vi "subvi_SerialRead.vi"(4 "tf_exit(Refnum)":refnum<vi>, 5 "Error In":errorcluster, 6 "error_out(Refnum)":refnum<vi>, 7 "baud_rate":u32=9600, 8 "tb_read_datetime(Refnum)":refnum<vi>, 9 "tb_read(Refnum)":refnum<vi>, 10 "tf_status(Refnum)":refnum<vi>, 11 "visa_device(Refnum)":refnum<vi>) -> ()   [LabVIEW 2019]
uses:
  <vilib>/Instr/_visa.llb/VISA Flush IO Buffer Mask.ctl
  <vilib>/Instr/_visa.llb/VISA Configure Serial Port (Instr).vi
panel:
  out "visa_device 2":refnum<visa-resource-name>
  out "error_out":errorcluster
  out "tb_read_datetime":string
  out "tb_read":string
  out "tf_exit_bool":bool
  in  "tf_exit":bool
  out "tf_status":bool
  in  "visa_device":refnum<visa-resource-name>
  # "Internal references"
  # "Controls used externally"
  # "External references"
  # "Controls used internally"
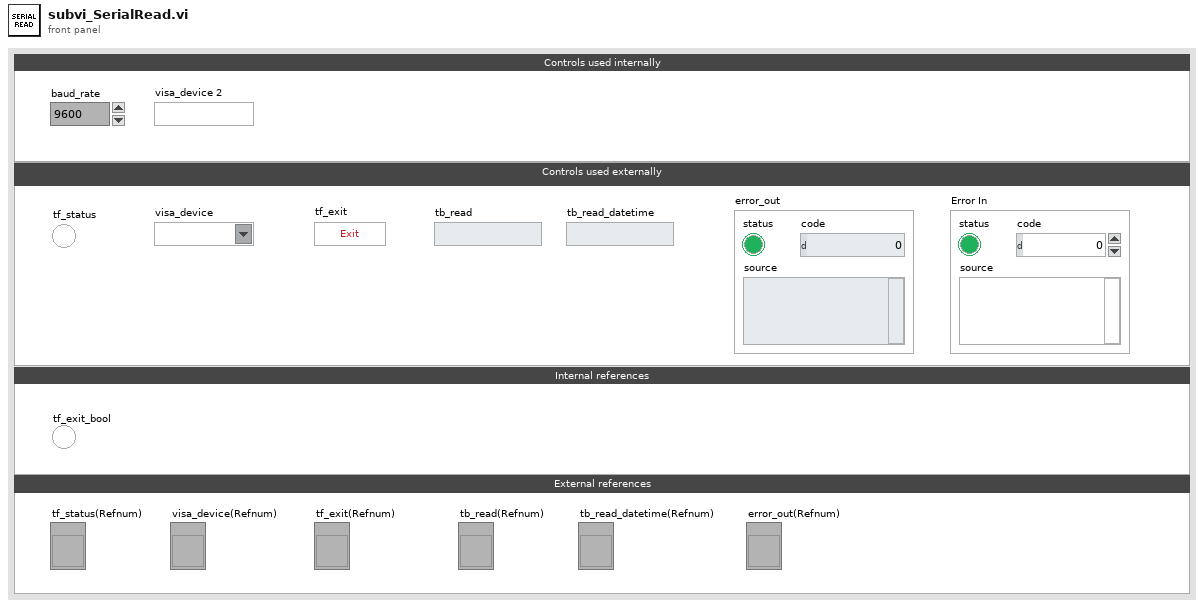
[diagram p1: front panel]
types:
  T1 = typedef "VISA Flush IO Buffer Mask.ctl" = u16
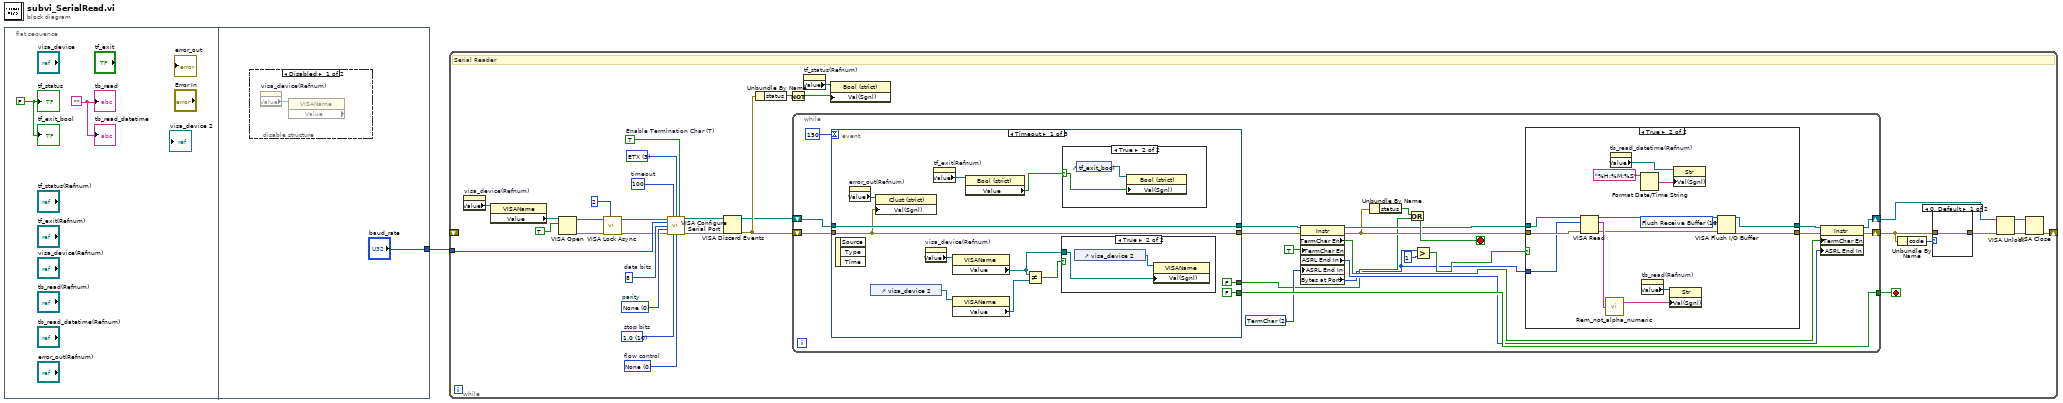
[diagram p0: block diagram]
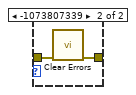
[diagram p3: hidden frame]
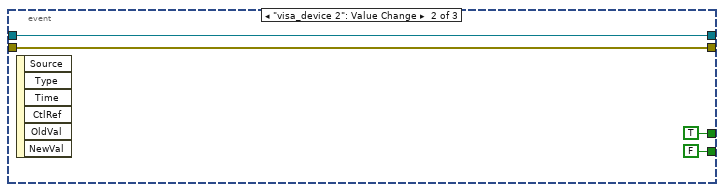
[diagram p6: hidden frame]
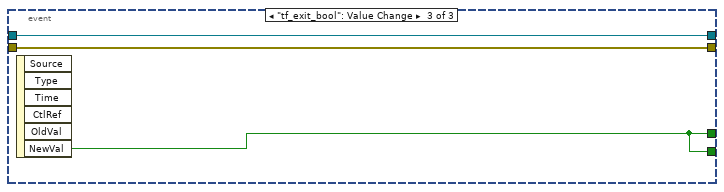
[diagram p7: hidden frame]
diagram:
  n1 = flat-sequence {
    tunnel: ["baud_rate"] -> w1
    frame #0 {
      w2 = ""
      w3 = FALSE ("tf_status")
      "tf_status" <- w3
      "tb_read" <- w2
      "tb_read_datetime" <- w2
      "tf_exit_bool" <- w3
    }
    frame #1 {
      n2 = disable-structure shown="Disabled" {
        frame Disabled {
          n3 = property on="visa_device(Refnum)" class="LVObjRef (strict)"() -> ("Value"=w5:refnum<vi>)  [unwired: 2 in, 2 out]
          n4 = property class="VISAName" props=["Value"](reference=w5) -> ()  [unwired: 1 in, 3 out]
        }
        frame Enabled {
        }
      }
    }
  }
  n5 = while {
    tunnel: w1 -> [w23]
    shift-right: [w21] -> _
    shift-left: _ -> [_]
    stop <- w28 stop-if-true
    w34 = u16 3 items=["LF"=10, "ETX"=3, "CR"=13] ("Sufix")
    w29 = u16 0 items=["None"=0, "XON/XOFF"=1, "RTS/CTS"=2, "DTR/DSR"=4]  # flow control
    w30 = u16 10 items=["1.0"=10, "1.5"=15, "2.0"=20]  # stop bits
    w31 = u16 0 items=["None", "Odd", "Even", "Mark", "Space"]  # parity
    w32 = u16 8  # data bits
    w35 = TRUE  # Enable Termination Char (T)
    w33 = u32 100  # timeout
    # "Serial Reader"
    n6 = property on="visa_device(Refnum)" class="LVObjRef (strict)"() -> ("Value"=w25:refnum<vi>)  [unwired: 2 in, 2 out]
    n7 = property class="VISAName"(reference=w25) -> ("Value"=w18:refnum<visa-resource-name>)  [unwired: 1 in, 2 out]
    n8 = VISA Open(duplicate session (F)=TRUE, VISA resource name=w18) -> (VISA resource name=w14:refnum<visa-resource-name>, error out=w13:errorcluster)  [unwired: 3 in]
    n9 = call <vilib>:"VISA Lock Async.vi"("lock type (exclusive: 1)"=u32 2, "error in (no error)"=w13, "VISA resource name"=w14) -> ("error out"=w11:errorcluster, "VISA resource name out"=w12:refnum<visa-resource-name>)  [unwired: 6 in, 1 out]
    n10 = call-poly "VISA Configure Serial Port"("VISA resource name"=w12, "timeout (10sec)"=w33, "termination char\n(0xA = '\\n' = LF)"=w34, "Enable Termination\nChar (T)"=w35, "baud rate (9600)"=w23, "data bits (8)"=w32, "parity (0:none)"=w31, "error in (no error)"=w11, "stop bits (10: 1 bit)"=w30, "flow control (0:none)"=w29) -> ("VISA resource name out"=w17:refnum<visa-resource-name>, "error out"=w16:errorcluster)  [unwired: 4 in]
    n11 = VISA Discard Events(8:w16, 11:w17) -> (0:w20:errorcluster, 3:w19:refnum<visa-resource-name>)  [unwired: 2 in]
    n12 = Unbundle By Name(w20) -> ("status"=w36:bool)
    n13 = Not(x=w36) -> (.not. x?=w26:bool)
    n14 = while {
      shift-right: [w58] -> w7
      shift-left: w19 -> [w61]
      shift-right: [w59] -> w22
      shift-left: w20 -> [w60]
      tunnel: [w56] -> w28
      stop <- w57 stop-if-true
      w47 = u16 2 items=["None", "Last Bit", "TermChar"] ("Serial Settings:End Mode for Reads")
      n15 = event shown="[0] Timeout" {
        selector: _ -> [_ _ _]
        dyn-events: _ -> [_ _ _]
        timeout: 150 -> [_ _ _]
        tunnel: [FALSE TRUE ("NewVal") w82] -> w41
        tunnel: [FALSE FALSE ("NewVal") w82] -> w56
        tunnel: w60 -> [w62 w78 w84]
        tunnel: w61 -> [w73 w79 w83]
        tunnel: [w73 w79 w83] -> w44
        tunnel: [w62 w78 w84] -> w43
        event Timeout {
          n16 = event-data() -> ()  [unwired: 1 in, 3 out]
          n17 = property on="error_out(Refnum)" class="LVObjRef (strict)"() -> ("Value"=w63:refnum<vi>)  [unwired: 2 in, 2 out]
          n18 = control-ref of="visa_device 2"() -> (w67:refnum<vi>)
          n19 = property on="Property Node" class="Clust (strict)"(reference=w63, "Val(Sgnl)"=w62) -> ()  [unwired: 1 in, 2 out]
          n20 = property on="visa_device(Refnum)" class="LVObjRef (strict)"() -> ("Value"=w69:refnum<vi>)  [unwired: 2 in, 2 out]
          n21 = property on="tf_exit(Refnum)" class="LVObjRef (strict)"() -> ("Value"=w70:refnum<vi>)  [unwired: 2 in, 2 out]
          n22 = property class="VISAName"(reference=w69) -> ("Value"=w64:refnum<visa-resource-name>)  [unwired: 1 in, 2 out]
          n23 = property class="VISAName"(reference=w67) -> ("Value"=w66:refnum<visa-resource-name>)  [unwired: 1 in, 2 out]
          n24 = property class="Bool (strict)"(reference=w70) -> ("Value"=w68:bool)  [unwired: 1 in, 2 out]
          n25 = Not Equal?(x=w64, y=w66) -> (x != y?=w65:bool)
          n26 = case shown="True" w65 {
            tunnel: w64 -> [_ w74]
            frame False {
            }
            frame True {
              n27 = control-ref of="visa_device 2"() -> (w75:refnum<vi>)
              n28 = property on="Property Node" class="VISAName"(reference=w75, "Val(Sgnl)"=w74) -> ()  [unwired: 1 in, 2 out]
            }
          }
          n29 = case shown="True" w68 {
            selector: w68 -> [_ w76]
            frame False {
            }
            frame True {
              n30 = control-ref of="tf_exit_bool"() -> (w77:refnum<vi>)
              n31 = property on="Property Node" class="Bool (strict)"(reference=w77, "Val(Sgnl)"=w76) -> ()  [unwired: 1 in, 2 out]
            }
          }
        }
        event "visa_device 2": Value Change {
          n32 = event-data() -> ()  [unwired: 1 in, 6 out]
        }
        event "tf_exit_bool": Value Change {
          n33 = event-data() -> ("NewVal"=w82:bool)  [unwired: 1 in, 5 out]
        }
      }
      n34 = property class="Instr"(reference=w44, error in=w43, "TermChar En"=TRUE, "ASRL End In"=w47) -> (reference out=w53:refnum<visa-resource-name>, error out=w52:errorcluster, "TermChar En"=w54:bool, "ASRL End In"=w55:u16, "Bytes at Port"=w40:u32)
      n35 = Unbundle By Name(w52) -> ("status"=w42:bool)
      n36 = Or(x=w42, y=w41) -> (x .or. y?=w57:bool)
      n37 = Greater?(x=w40, y=u32 1) -> (0:w49:bool)
      n38 = case shown="True" w49 {
        tunnel: [w86 w88] -> w51
        tunnel: [w85 w87] -> w50
        tunnel: w53 -> [w86 w98]
        tunnel: w52 -> [w85 w97]
        tunnel: w40 -> [_ w92]
        frame False {
        }
        frame True {
          w91 = T1 16 items=["Flush Receive Buffer"=16, "Write Transmit Buffer to Device"=32, "Flush Receive Buffer (No I/O)"=64, "Flush Transmit Buffer"=128] ("Mask")
          n39 = VISA Read(VISA resource name=w98, byte count=w92, error in (no error)=w97) -> (VISA resource name out=w90:refnum<visa-resource-name>, read buffer=w100:string, error out=w89:errorcluster)  [unwired: 1 out]
          n40 = call "Rem_not_alpha_numeric.vi"("In_String"=w100) -> ("clan_String"=w99:string)  [unwired: 1 out]
          n41 = property on="tb_read_datetime(Refnum)" class="LVObjRef (strict)"() -> ("Value"=w93:refnum<vi>)  [unwired: 2 in, 2 out]
          n42 = Format Date/Time String(time format string (%c)="%H:%M:%S") -> (date/time string=w96:string)  [unwired: 2 in]
          n43 = property on="tb_read(Refnum)" class="LVObjRef (strict)"() -> ("Value"=w94:refnum<vi>)  [unwired: 2 in, 2 out]
          n44 = property on="Property Node" class="Str"(reference=w94, "Val(Sgnl)"=w99) -> ()  [unwired: 1 in, 2 out]
          n45 = property on="Property Node" class="Str"(reference=w93, "Val(Sgnl)"=w96) -> ()  [unwired: 1 in, 2 out]
          n46 = VISA Flush I/O Buffer(VISA resource name=w90, mask (16)=w91, error in (no error)=w89) -> (VISA resource name out=w88:refnum<visa-resource-name>, error out=w87:errorcluster)
        }
      }
      n47 = property class="Instr"(reference=w51, error in=w50, "TermChar En"=w54, "ASRL End In"=w55) -> (reference out=w58:refnum<visa-resource-name>, error out=w59:errorcluster)
    }
    n48 = property on="tf_status(Refnum)" class="LVObjRef (strict)"() -> ("Value"=w24:refnum<vi>)  [unwired: 2 in, 2 out]
    n49 = property on="Property Node" class="Bool (strict)"(reference=w24, "Val(Sgnl)"=w26) -> ()  [unwired: 1 in, 2 out]
    n50 = Unbundle By Name(w22) -> ("code"=w27:i32)
    n51 = case shown="0, Default" w27 {
      tunnel: w22 -> [w37 w39]
      tunnel: [w37 w38] -> w8
      frame 0, Default {
      }
      frame -1073807339 {
        n52 = call <vilib>:"Clear Errors.vi"("error in (no error)"=w39) -> ("error out"=w38:errorcluster)  [unwired: 5 in, 1 out]
      }
    }
    n53 = VISA Unlock(8:w8, 11:w7) -> (0:w9:errorcluster, 3:w6:refnum<visa-resource-name>)
    n54 = VISA Close(VISA resource name=w6, error in (no error)=w9) -> (error out=w21:errorcluster)
  }
